vi "Instantaneous Lag.vi"(8 "error in (no error)":errorcluster, 9 "Instant Stimulus Value":dbl, 10 "Instant (sample)":dbl, 11 "Response Polynomial Coefficients":dbl[](array[numeric])) -> (0 "error out":errorcluster, 3 "Instant Response Lag (sample)":dbl)   [LabVIEW 2014, in "Head Impulse Fit.lvclass"]
uses:
  Head Impulse Fit.lvclass
  <vilib>/Analysis/polynomials.llb/Add Polynomials (DBL).vi
  <vilib>/Analysis/polynomials.llb/Polynomial Roots (DBL).vi
  <userlib>/_OpenG.lib/array/array.llb/Conditional Auto-Indexing Tunnel (DBL)__ogtk.vi
  <userlib>/_OpenG.lib/array/array.llb/Sort 1D Array (DBL)__ogtk.vi
  <vilib>/Analysis/NI_AALPro.lvlib
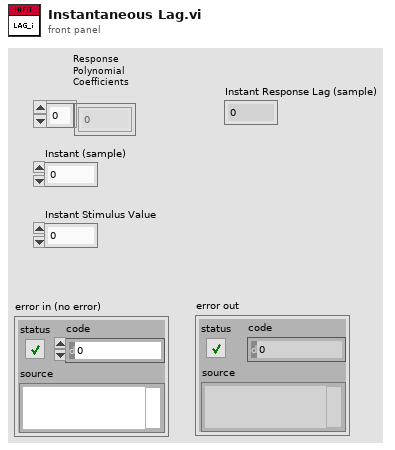
[diagram p1: front panel]
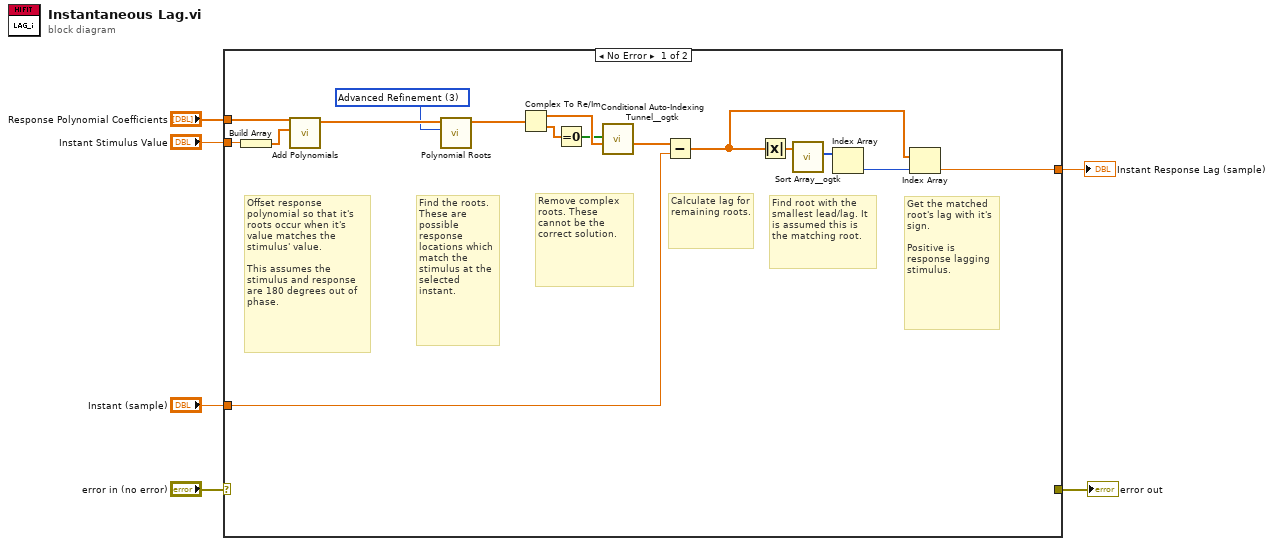
[diagram p0: block diagram]
diagram:
  n1 = case shown="No Error" "error in (no error)" {
    selector: "error in (no error)" -> [_ w23]
    tunnel: "Response Polynomial Coefficients" -> [w22 _]
    tunnel: "Instant Stimulus Value" -> [w21 _]
    tunnel: "Instant (sample)" -> [w12 _]
    tunnel: [w7 _] -> w2
    tunnel: [_ w23] -> w1
    frame No Error {
      w18 = u16 3 items=["General", "Simple Classification", "Refinement", "Advanced Refinement"] ("option")
      # "Get the matched root's lag with it's sign.\n\nPositive is response lagging stimulus."
      # "Calculate lag for remaining roots."
      # "Find root with the smallest lead/lag. It is assumed this is the matching root."
      # "Remove complex roots. These cannot be the correct solution."
      # "Find the roots. These are possible response locations which match the stimulus at the selected instant."
      # "Offset response polynomial so that it's roots occur when it's value matches the stimulus' value.\n\nThis assumes the stimulus and response are 180 degrees out of phase."
      n2 = Build Array(w21) -> (w20:dbl[])
      n3 = call-poly <vilib>:"Add Polynomials.vi"("Q(x)"=w20, "P(x)"=w22) -> ("P(x)+Q(x)"=w19:dbl[])  [unwired: 8 in, 1 out]
      n4 = call-poly <vilib>:"Polynomial Roots.vi"("option"=w18, "P(x)"=w19) -> ("Roots"=w17:cdb[])  [unwired: 8 in, 1 out]
      n5 = Complex To Re/Im(x + iy=w17) -> (x=w15:dbl[], y=w16:dbl[])
      n6 = Equal To 0?(x=w16) -> (x = 0?=w14:bool[])
      n7 = call-poly <userlib>:"Conditional Auto-Indexing Tunnel__ogtk.vi"("Array in"=w15, "Elements to keep"=w14) -> ("Filtered Array out"=w13:dbl[])  [unwired: 5 in]
      n8 = Subtract(x=w13, y=w12) -> (x-y=w9:dbl[])
      n9 = Absolute Value(x=w9) -> (abs(x)=w10:dbl[])
      n10 = call-poly <userlib>:"Sort Array__ogtk.vi"("Array in"=w10) -> ("Sorted Pointers"=w11:i32[])  [unwired: 9 in, 1 out]
      n11 = Index Array(array=w11) -> (element=w8:i32)  [unwired: 1 in]
      n12 = Index Array(array=w9, index=w8) -> (element=w7:dbl)
    }
    frame Error {
    }
  }
  "error out" <- w1
  "Instant Response Lag (sample)" <- w2
